vi "ButtonPickupNextTote.vi"(11 "Buttons":bool[](array[boolean])) -> ()   [LabVIEW 2014]
uses:
  LowerLiftAndOpenArms.ctl
  Gantry/GantryGlobals.vi
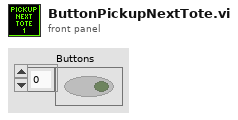
[diagram p1: front panel]
types:
  T1 = typedef "LowerLiftAndOpenArms.ctl" = enum16{"WaitingForInput", "LowerLift", "OpenArms", "LowerLiftMore", "CloseArms", "RaiseLift", "StopArms"}
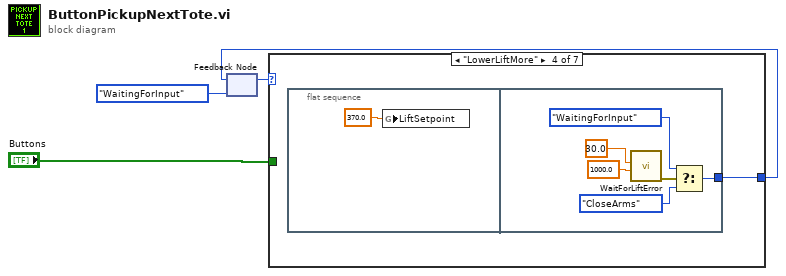
[diagram p0: block diagram]
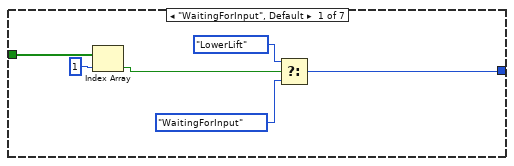
[diagram p2: hidden frame]
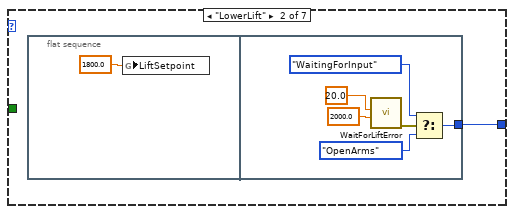
[diagram p3: hidden frame]
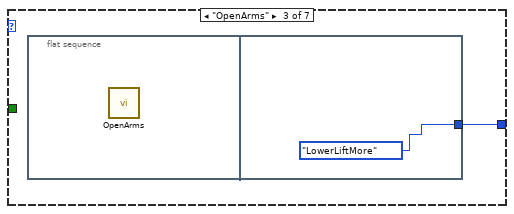
[diagram p4: hidden frame]
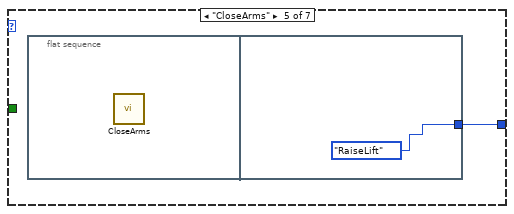
[diagram p5: hidden frame]
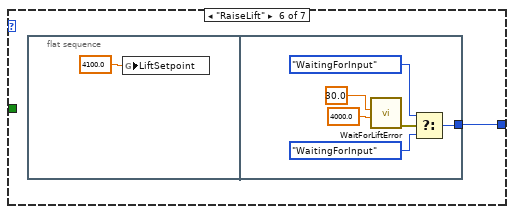
[diagram p6: hidden frame]
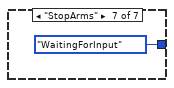
[diagram p7: hidden frame]
diagram:
  n1 = feedback #1(LowerLiftAndOpenArms."WaitingForInput" ("LowerAndOpen")) -> (w2:T1)
  n2 = case shown="\"LowerLiftMore\"" w2 {
    tunnel: [w7 w11 w19 w21 w29 w31 LowerLiftAndOpenArms."WaitingForInput" ("LowerAndOpen")] -> w1
    tunnel: "Buttons" -> [w6 _ _ _ _ _ _]
    frame "WaitingForInput", Default {
      n3 = Index Array(array=w6, index=1) -> (element=w5:bool)
      n4 = Select(t=LowerLiftAndOpenArms."LowerLift" ("LowerAndOpen"), s=w5, f=LowerLiftAndOpenArms."WaitingForInput" ("LowerAndOpen")) -> (s? t:f=w7:T1)
    }
    frame "LowerLift" {
      n5 = flat-sequence {
        tunnel: [w13] -> w11
        frame #0 {
          n6 = global write "GantryGlobals.vi" "LiftSetpoint"(1800.0 ("LiftSetpoint")) -> ()
        }
        frame #1 {
          n7 = call "WaitForLiftError.vi"("Timeout (ms)"=2000.0, "AllowedError"=20.0) -> ("error out"=w16:errorcluster)  [unwired: 9 in]
          n8 = Select(t=LowerLiftAndOpenArms."WaitingForInput" ("LowerAndOpen"), s=w16, f=LowerLiftAndOpenArms."OpenArms" ("LowerAndOpen")) -> (s? t:f=w13:T1)
        }
      }
    }
    frame "OpenArms" {
      n9 = flat-sequence {
        tunnel: [LowerLiftAndOpenArms."LowerLiftMore" ("LowerAndOpen")] -> w19
        frame #0 {
          n10 = call "OpenArms.vi"() -> ()  [unwired: 12 in]
        }
        frame #1 {
        }
      }
    }
    frame "LowerLiftMore" {
      n11 = flat-sequence {
        tunnel: [w23] -> w21
        frame #0 {
          n12 = global write "GantryGlobals.vi" "LiftSetpoint"(370.0 ("LiftSetpoint")) -> ()
        }
        frame #1 {
          n13 = call "WaitForLiftError.vi"("Timeout (ms)"=1000.0, "AllowedError"=30.0) -> ("error out"=w26:errorcluster)  [unwired: 9 in]
          n14 = Select(t=LowerLiftAndOpenArms."WaitingForInput" ("LowerAndOpen"), s=w26, f=LowerLiftAndOpenArms."CloseArms" ("LowerAndOpen")) -> (s? t:f=w23:T1)
        }
      }
    }
    frame "CloseArms" {
      n15 = flat-sequence {
        tunnel: [LowerLiftAndOpenArms."RaiseLift" ("LowerAndOpen")] -> w29
        frame #0 {
          n16 = call "CloseArms.vi"() -> ()  [unwired: 12 in]
        }
        frame #1 {
        }
      }
    }
    frame "RaiseLift" {
      n17 = flat-sequence {
        tunnel: [w33] -> w31
        frame #0 {
          n18 = global write "GantryGlobals.vi" "LiftSetpoint"(4100.0 ("LiftSetpoint")) -> ()
        }
        frame #1 {
          n19 = call "WaitForLiftError.vi"("Timeout (ms)"=4000.0, "AllowedError"=30.0) -> ("error out"=w36:errorcluster)  [unwired: 9 in]
          n20 = Select(t=LowerLiftAndOpenArms."WaitingForInput" ("LowerAndOpen"), s=w36, f=LowerLiftAndOpenArms."WaitingForInput" ("LowerAndOpen")) -> (s? t:f=w33:T1)
        }
      }
    }
    frame "StopArms" {
    }
  }
  n21 = feedback-in #1(w1) -> ()
